vi "Close Device Core.vi"(8 "error in (no error)":errorcluster, 11 "BNT_ULx-MCSV in":refnum<class "BNT_ULx-MCSV.lvclass">) -> (0 "error out":errorcluster, 3 "BNT_ULx-MCSV out":refnum<class "BNT_ULx-MCSV.lvclass">)   [LabVIEW 2020, in "BNT_ULx.lvlib" / "BNT_ULx-MCSV.lvclass"]
doc: "Close device driver connection."
uses:
  BNT_ULx-MCSV.lvclass
  BNT_ULx-MCSV.lvclass/BNT_ULx-MCSV.ctl
  CSPP_Core/Actors/CSPP_DeviceActor/CSPP_DeviceActor.lvclass
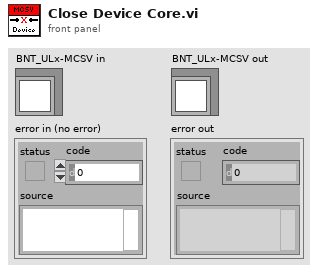
[diagram p1: front panel]
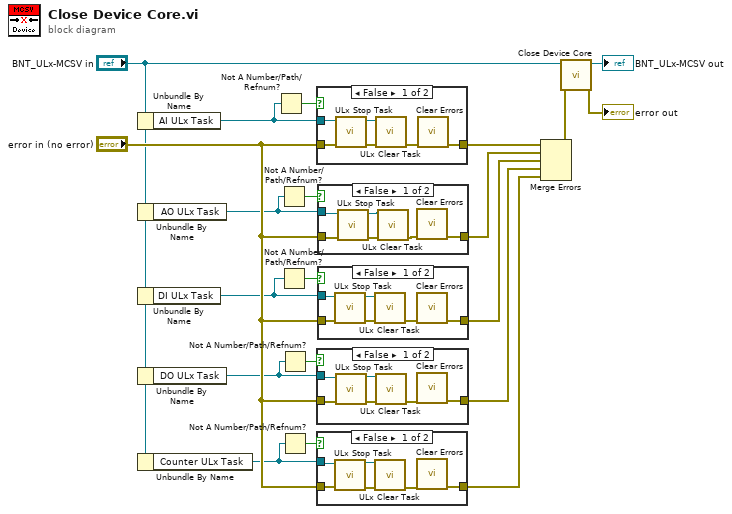
[diagram p0: block diagram]
diagram:
  n1 = Unbundle By Name("BNT_ULx-MCSV in") -> ("AI ULx Task"=w10:refnum<k24>)
  n2 = Unbundle By Name("BNT_ULx-MCSV in") -> ("AO ULx Task"=w7:refnum<k24>)
  n3 = Unbundle By Name("BNT_ULx-MCSV in") -> ("DI ULx Task"=w5:refnum<k24>)
  n4 = Unbundle By Name("BNT_ULx-MCSV in") -> ("DO ULx Task"=w3:refnum<k24>)
  n5 = Unbundle By Name("BNT_ULx-MCSV in") -> ("Counter ULx Task"=w1:refnum<k24>)
  n6 = Not A Number/Path/Refnum?(number/path/refnum=w10) -> (NaN/Path/Refnum?=w9:bool)
  n7 = Not A Number/Path/Refnum?(number/path/refnum=w7) -> (NaN/Path/Refnum?=w8:bool)
  n8 = Not A Number/Path/Refnum?(number/path/refnum=w5) -> (NaN/Path/Refnum?=w6:bool)
  n9 = Not A Number/Path/Refnum?(number/path/refnum=w3) -> (NaN/Path/Refnum?=w4:bool)
  n10 = Not A Number/Path/Refnum?(number/path/refnum=w1) -> (NaN/Path/Refnum?=w2:bool)
  n11 = case shown="False" w9 {
    tunnel: [w26 w27] -> w18
    tunnel: "error in (no error)" -> [w24 w27]
    tunnel: w10 -> [w25 _]
    frame False {
      n12 = call <vilib>:"ULx Stop Task.vi"("error in"=w24, "task in"=w25) -> ("error out"=w22:errorcluster, "task out"=w23:refnum<k24>)  [unwired: 8 in]
      n13 = call <vilib>:"ULx Clear Task.vi"("task in"=w23, "error in"=w22) -> ("error out"=w21:errorcluster)  [unwired: 13 in]
      n14 = call <vilib>:"Clear Errors.vi"("error in (no error)"=w21) -> ("error out"=w26:errorcluster)  [unwired: 5 in, 1 out]
    }
    frame True {
    }
  }
  n15 = case shown="False" w4 {
    tunnel: w3 -> [w29 _]
    tunnel: [w33 w34] -> w14
    tunnel: "error in (no error)" -> [w31 w34]
    frame False {
      n16 = call <vilib>:"ULx Stop Task.vi"("error in"=w31, "task in"=w29) -> ("error out"=w32:errorcluster, "task out"=w28:refnum<k24>)  [unwired: 8 in]
      n17 = call <vilib>:"ULx Clear Task.vi"("task in"=w28, "error in"=w32) -> ("error out"=w30:errorcluster)  [unwired: 13 in]
      n18 = call <vilib>:"Clear Errors.vi"("error in (no error)"=w30) -> ("error out"=w33:errorcluster)  [unwired: 5 in, 1 out]
    }
    frame True {
    }
  }
  n19 = case shown="False" w2 {
    tunnel: w1 -> [w35 _]
    tunnel: "error in (no error)" -> [w38 w41]
    tunnel: [w40 w41] -> w12
    frame False {
      n20 = call <vilib>:"ULx Stop Task.vi"("error in"=w38, "task in"=w35) -> ("error out"=w39:errorcluster, "task out"=w36:refnum<k24>)  [unwired: 8 in]
      n21 = call <vilib>:"ULx Clear Task.vi"("task in"=w36, "error in"=w39) -> ("error out"=w37:errorcluster)  [unwired: 13 in]
      n22 = call <vilib>:"Clear Errors.vi"("error in (no error)"=w37) -> ("error out"=w40:errorcluster)  [unwired: 5 in, 1 out]
    }
    frame True {
    }
  }
  n23 = case shown="False" w8 {
    tunnel: w7 -> [w43 _]
    tunnel: [w47 w48] -> w16
    tunnel: "error in (no error)" -> [w45 w48]
    frame False {
      n24 = call <vilib>:"ULx Stop Task.vi"("error in"=w45, "task in"=w43) -> ("error out"=w46:errorcluster, "task out"=w42:refnum<k24>)  [unwired: 8 in]
      n25 = call <vilib>:"ULx Clear Task.vi"("task in"=w42, "error in"=w46) -> ("error out"=w44:errorcluster)  [unwired: 13 in]
      n26 = call <vilib>:"Clear Errors.vi"("error in (no error)"=w44) -> ("error out"=w47:errorcluster)  [unwired: 5 in, 1 out]
    }
    frame True {
    }
  }
  n27 = case shown="False" w6 {
    tunnel: w5 -> [w51 _]
    tunnel: [w54 w55] -> w15
    tunnel: "error in (no error)" -> [w52 w55]
    frame False {
      n28 = call <vilib>:"ULx Stop Task.vi"("error in"=w52, "task in"=w51) -> ("error out"=w53:errorcluster, "task out"=w50:refnum<k24>)  [unwired: 8 in]
      n29 = call <vilib>:"ULx Clear Task.vi"("task in"=w50, "error in"=w53) -> ("error out"=w49:errorcluster)  [unwired: 13 in]
      n30 = call <vilib>:"Clear Errors.vi"("error in (no error)"=w49) -> ("error out"=w54:errorcluster)  [unwired: 5 in, 1 out]
    }
    frame True {
    }
  }
  n31 = Merge Errors(w18, w16, w15, w14, w12) -> (w17:errorcluster)
  n32 = call-parent "Close Device Core.vi"("error in (no error)"=w17, "CSPP_DeviceActor in"="BNT_ULx-MCSV in") -> ("error out"=→"error out":errorcluster, "CSPP_DeviceActor out"=→"BNT_ULx-MCSV out":refnum<class "BNT_ULx-MCSV.lvclass">)  [unwired: 8 in]
